vi "Get Sensor Mode.vi"(8 "error in (no error)":errorcluster, 11 "hdl in":i32) -> (0 "error out":errorcluster, 2 "Get Sensor Mode":T1(ring), 3 "hdl out":i32)   [LabVIEW 2013, in "Thorlabs_FWxC.lvlib"]
uses:
  <instrlib>/Thorlabs_FWxC/Thorlabs_FWxC.lvlib
  <instrlib>/Thorlabs_FWxC/Library/FilterWheel102_win32.dll
  <instrlib>/Thorlabs_FWxC/Library/FilterWheel102_win64.dll
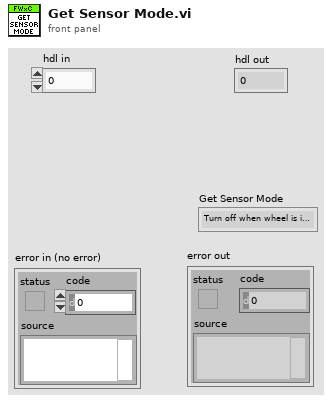
[diagram p1: front panel]
types:
  T1 = enum16{"Turn off when wheel is idle to eliminate stray light", "Remain active"}
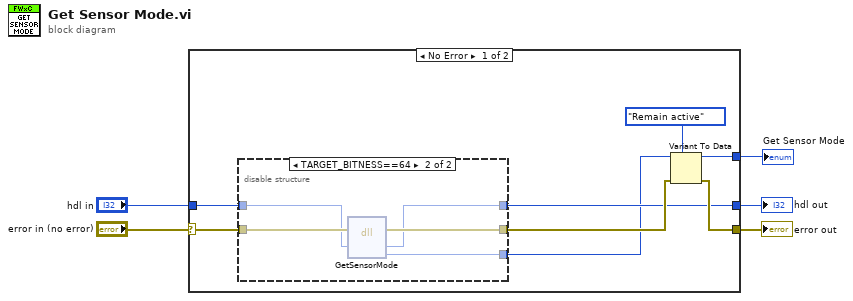
[diagram p0: block diagram]
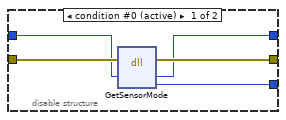
[diagram p2: hidden frame]
diagram:
  n1 = case shown="No Error" "error in (no error)" {
    selector: "error in (no error)" -> [w10 w24]
    tunnel: [w12 w24] -> w5
    tunnel: "hdl in" -> [w8 w25]
    tunnel: [w7 w25] -> w2
    tunnel: [w13 _] -> w1
    frame No Error {
      n2 = disable-structure shown="TARGET_BITNESS==64" {
        disable-tunnel: w10 -> [w18 w23]
        disable-tunnel: [w17 w22] -> w9
        disable-tunnel: w8 -> [w16 w21]
        disable-tunnel: [w15 w20] -> w7
        disable-tunnel: [w14 w19] -> w6
        frame condition #0 (active) {
          n3 = dll-call lib="C:/Program Files (x86)/National Instruments/LabVIEW 2013/instr.lib/Thorlabs_FWxC/Library/FilterWheel102_win32.dll" fn="GetSensorMode"(error in=w18, "hdl"=w16) -> (error out=w17:errorcluster, "hdl"=w15:i32, "sensor mode"=w14:i32)  [unwired: 4 in, 1 out]
        }
        frame condition #1 {
          n4 = dll-call lib="C:/Program Files/National Instruments/LabVIEW 2013/instr.lib/Thorlabs_FWxC/Library/FilterWheel102_win64.dll" fn="GetSensorMode"(error in=w23, "hdl"=w21) -> (error out=w22:errorcluster, "hdl"=w20:i32, "sensor mode"=w19:i32)  [unwired: 4 in, 1 out]
        }
      }
      n5 = Variant To Data(error in=w9, type=T1."Remain active" ("Sensor Mode"), Variant=w6) -> (data=w13:T1, error out=w12:errorcluster)
    }
    frame Error {
    }
  }
  "error out" <- w5
  "hdl out" <- w2
  "Get Sensor Mode" <- w1
